vi "createBroadcastStepMotorFrame.vi"(8 "error in (no error)":errorcluster, 10 "BroadcastCounter":u8, 11 "HardPointActuator in":refnum<class "HPILC.lvclass">) -> (0 "error out":errorcluster, 2 "FixedFrameBuilder":refnum<class "FixedFrameBuilder.lvclass">, 3 "HardPointActuator out":refnum<class "HPILC.lvclass">)   [LabVIEW 2015, in "RTHPILC.lvlib" / "HPILC.lvclass"]
uses:
  HPILC.lvclass
  Common_RT_Modbus/FixedFrameBuilder/FixedFrameBuilder.lvclass
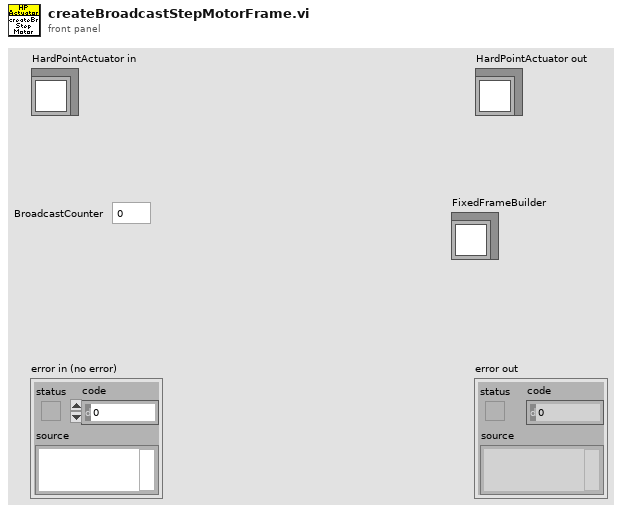
[diagram p1: front panel]
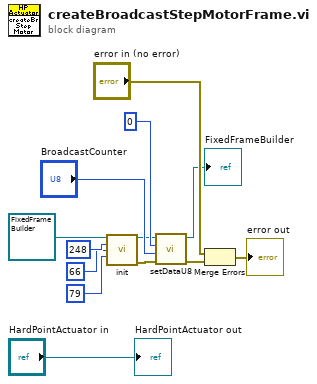
[diagram p0: block diagram]
diagram:
  n1 = call "init.vi"("FixedFrameBuilder in"=refnum<class "FixedFrameBuilder.lvclass"> refnum ("RTModbus.lvlib:FixedFrameBuilder.lvclass"), "Address"=u8 248, "Function"=u8 66, "DataSize"=79) -> ("FixedFrameBuilder out"=w3:refnum<class "FixedFrameBuilder.lvclass">, "error out"=w4:errorcluster)  [unwired: 10 in]
  n2 = call "setDataU8.vi"("error in (no error)"=w4, "Data"="BroadcastCounter", "Index"=0, "FixedFrameBuilder in"=w3) -> ("error out"=w1:errorcluster, "FixedFrameBuilder out"=→"FixedFrameBuilder":refnum<class "FixedFrameBuilder.lvclass">)  [unwired: 6 in]
  n3 = Merge Errors("error in (no error)", w1) -> (→"error out":errorcluster)
  "HardPointActuator out" <- "HardPointActuator in"
